vi "CS상태머신서버장난감.vi"() -> ()   [LabVIEW 2018]
uses:
  <vilib>/LabVIEW Open Source Project/Connection/Connection/Connection.lvclass
  <vilib>/LabVIEW Open Source Project/MQTT TCP Connection/MQTT_TCP/Connection/TCPConnection.lvclass
  C:/Program Files (x86)/National Instruments/LabVIEW 2018/vi.lib/LabVIEW Open Source Project/Connection/Connection/Connection.lvclass
panel:
  in  "파일 경로(대화 상자 사용)":path
  out "All Files in Dir":path[](array[path]) caption="디렉토리내의 모든 파일"
  out "문자열":string
  out "listener error":errorcluster
  out "server session error":errorcluster
  out "client connected":bool
  in  "정지":bool
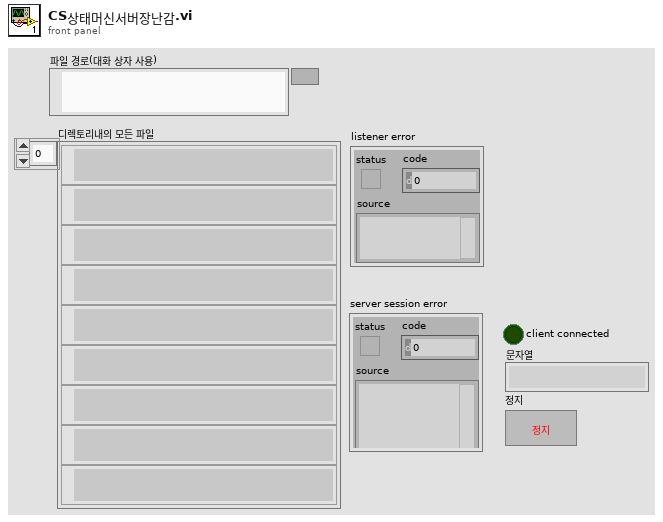
[diagram p1: front panel]
types:
  T1 = typedef "장난감컨트롤.ctl" = enum16{"대기", "연결됨", "연결종료", "종료", "업데이트", "다운로드"}
  T2 = enum16{"open", "replace", "create", "open or create", "replace or create", "replace or create with confirmation"}
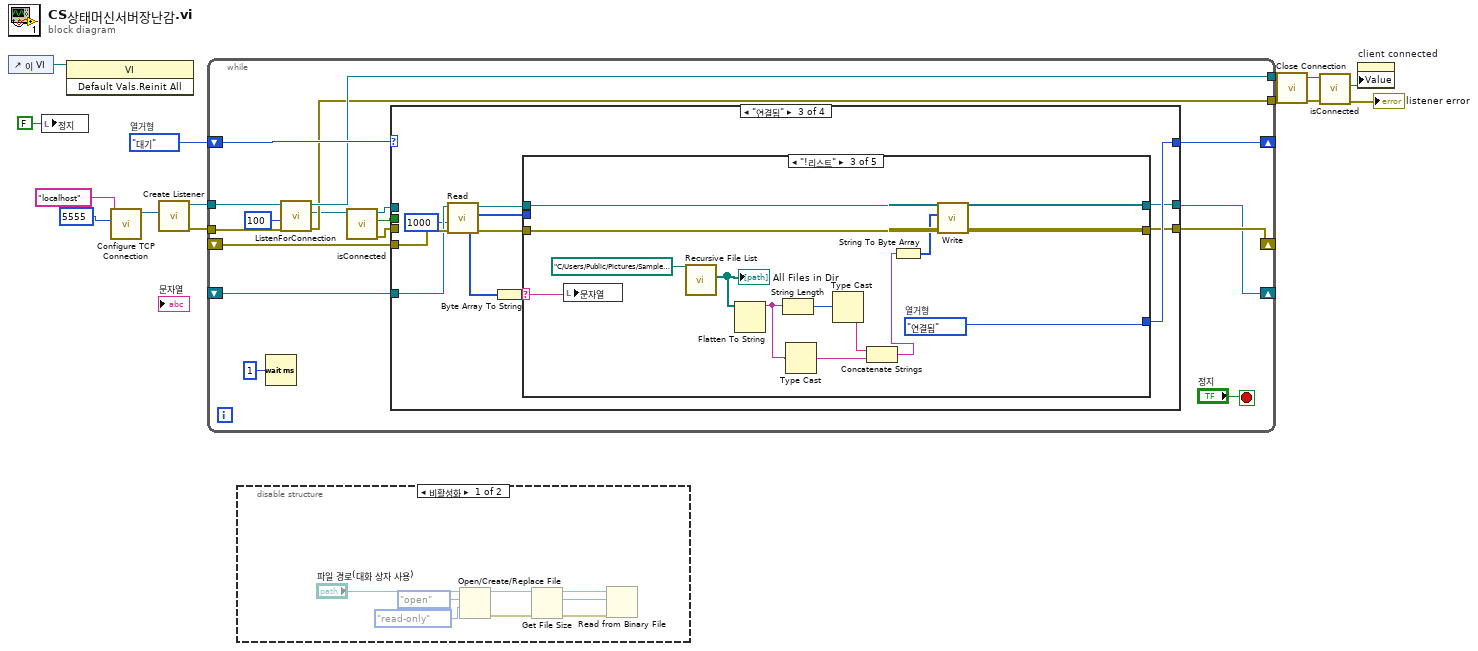
[diagram p0: block diagram]
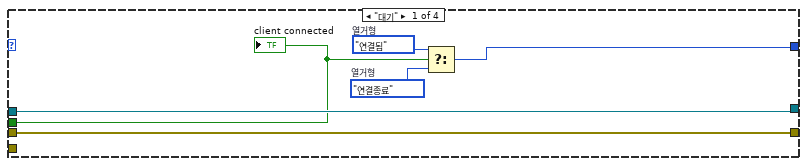
[diagram p3: hidden frame]
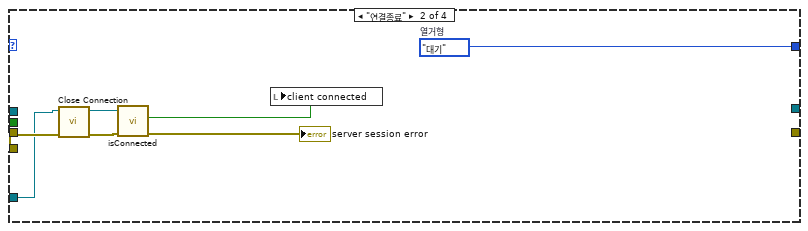
[diagram p4: hidden frame]
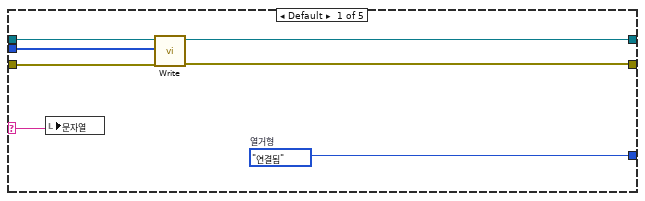
[diagram p5: hidden frame]
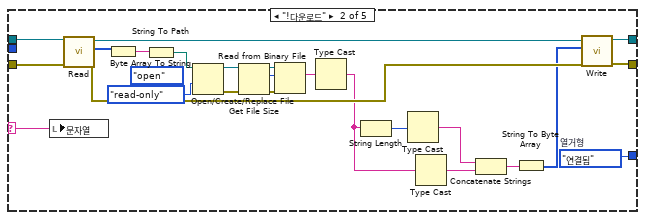
[diagram p6: hidden frame]
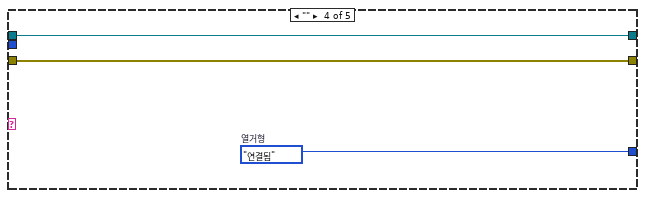
[diagram p7: hidden frame]
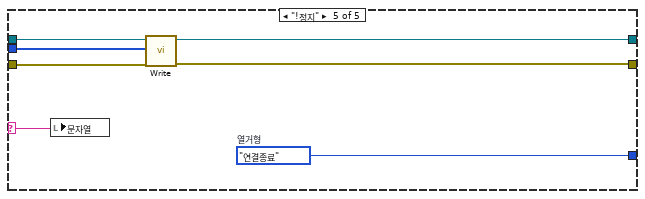
[diagram p8: hidden frame]
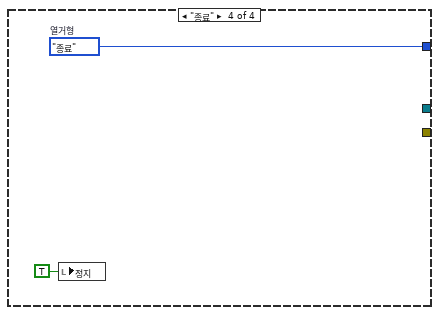
[diagram p9: hidden frame]
diagram:
  w7 = 장난감컨트롤."대기"  # 열거형
  n1 = control-ref of="이 VI"() -> (w11:refnum<vi>)
  n2 = local write "정지"(FALSE ("정지")) -> ()
  n3 = invoke class="VI" method="Default Vals.Reinit All"(reference=w11) -> ()  [unwired: 2 in, 3 out]
  n4 = call <vilib>:"Configure TCP Connection.vi"("remote port (80)"=u16 5555, "address (localhost)"="localhost") -> ("TCPConnection"=w14:refnum<class "TCPConnection.lvclass">)  [unwired: 8 in, 1 out]
  n5 = call <vilib>:"Create Listener.vi"("Connection Configuration"=w14) -> ("error out"=w6:errorcluster, "Listener"=w5:refnum<class "TCPConnection.lvclass">)  [unwired: 9 in]
  n6 = while {
    tunnel: [w27] -> w9
    tunnel: [w25] -> w8
    shift-right: [w28] -> _
    shift-left: w7 -> [w29]
    tunnel: w6 -> [w26]
    shift-right: [w24] -> _
    shift-left: _ -> [w23]
    tunnel: w5 -> [w17]
    shift-right: [w16] -> _
    shift-left: _ -> [w15]
    stop <- "정지" stop-if-true
    n7 = Wait (ms)(milliseconds to wait=u32 1 ("대기 시간 (ms)")) -> ()  [unwired: 1 out]
    n8 = call <vilib>:"ListenForConnection.vi"("error in (no error)"=w26, "timeout (2000 ms)"=100, "Listener"=w17) -> ("error out"=w25:errorcluster, "Connection"=w22:refnum<class "Connection.lvclass">, "Listener out"=w27:refnum<class "TCPConnection.lvclass">)  [unwired: 5 in, 1 out]
    n9 = call <vilib>:"isConnected.vi"("Connection in"=w22) -> ("error out"=w20:errorcluster, "connected"=w19:bool, "Connection out"=w21:refnum<class "Connection.lvclass">)  [unwired: 8 in]
    n10 = case shown="\"연결됨\"" w29 {
      tunnel: [w37 w40 w50 w111] -> w28
      tunnel: [w34 _ w46 _] -> w16
      tunnel: [w32 _ w45 _] -> w24
      tunnel: w23 -> [_ w39 w54 _]
      tunnel: w21 -> [w34 _ _ _]
      tunnel: w20 -> [w32 _ _ _]
      tunnel: w19 -> [w33 _ _ _]
      tunnel: w15 -> [_ w38 w53 _]
      frame "대기" {
        w35 = 장난감컨트롤."연결종료"  # 열거형
        w36 = 장난감컨트롤."연결됨"  # 열거형
        n11 = Select(t=w36, s=w33, f=w35) -> (s? t:f=w37:T1)
        "client connected" <- w33
      }
      frame "연결종료" {
        w40 = 장난감컨트롤."대기"  # 열거형
        n12 = call <vilib>:"Close Connection.vi"("error in (no error)"=w39, "Connection in"=w38) -> ("error out"=w41:errorcluster, "No Connection"=w43:refnum<class "Connection.lvclass">)  [unwired: 8 in]
        n13 = call <vilib>:"isConnected.vi"("error in (no error)"=w41, "Connection in"=w43) -> ("error out"=→"server session error":errorcluster, "connected"=w44:bool)  [unwired: 7 in, 1 out]
        n14 = local write "client connected"(w44) -> ()
      }
      frame "연결됨" {
        n15 = call <vilib>:"Read.vi"("error in (no error)"=w54, "timeout (2000 ms)"=1000, "TCPConnection in"=w53) -> ("error out"=w49:errorcluster, "Bytes"=w48:u8[], "TCPConnection out"=w47:refnum<class "Connection.lvclass">)  [unwired: 4 in, 2 out]
        n16 = Byte Array To String(unsigned byte array=w48) -> (string=w51:string)
        n17 = case shown="\"!리스트\"" w51 {
          selector: w51 -> [w61 w66 w99 _ w103]
          tunnel: [w60 w71 w98 w102 w109] -> w50
          tunnel: w49 -> [w59 w84 w97 w100 w106]
          tunnel: w48 -> [w58 _ _ _ w107]
          tunnel: w47 -> [w57 w85 w96 w101 w108]
          tunnel: [w56 w73 w95 w101 w104] -> w46
          tunnel: [w55 w72 w94 w100 w105] -> w45
          frame Default {
            w60 = 장난감컨트롤."연결됨"  # 열거형
            n18 = local write "문자열"(w61) -> ()
            n19 = call <vilib>:"Write.vi"("error in (no error)"=w59, "Bytes"=w58, "Connection in"=w57) -> ("error out"=w55:errorcluster, "Connection"=w56:refnum<class "Connection.lvclass">)  [unwired: 7 in]
          }
          frame "!다운로드" {
            w71 = 장난감컨트롤."연결됨"  # 열거형
            (unwired) T2."open" ("동작(0:open)")
            n20 = local write "문자열"(w66) -> ()
            n21 = call <vilib>:"Read.vi"("error in (no error)"=w84, "TCPConnection in"=w85) -> ("error out"=w74:errorcluster, "Bytes"=w83:u8[], "TCPConnection out"=w75:refnum<class "Connection.lvclass">)  [unwired: 5 in, 2 out]
            n22 = Byte Array To String(unsigned byte array=w83) -> (string=w79:string)
            n23 = String To Path(string=w79) -> (path=w78:path)
            n24 = Open/Create/Replace File(file path (use dialog)=w78, access (0:read/write)=enum16{"read/write", "read-only", "write-only"}."read-only" ("접근(0:읽기/쓰기)")) -> (refnum out=w77:refnum<file>, error out=w81:errorcluster)  [unwired: 4 in, 1 out]
            n25 = Get File Size(file=w77, error in=w81) -> (refnum out=w76:refnum<file>, size (in bytes)=w65:i64, 0:w82:errorcluster)
            n26 = Read from Binary File(8:w82, 10:w65, 11:w76) -> (2:w64:string)  [unwired: 3 in, 3 out]
            n27 = Type Cast(x=w64) -> (*(type *) &x=w62:string)  [unwired: 1 in]
            n28 = String Length(string=w62) -> (length=w63:i32)
            n29 = Type Cast(x=w63) -> (*(type *) &x=w70:string)  [unwired: 1 in]
            n30 = Type Cast(x=w62) -> (*(type *) &x=w69:string)  [unwired: 1 in]
            n31 = Concatenate Strings(w70, w69) -> (w68:string)
            n32 = String To Byte Array(string=w68) -> (unsigned byte array=w67:u8[])
            n33 = call <vilib>:"Write.vi"("error in (no error)"=w74, "Bytes"=w67, "Connection in"=w75) -> ("error out"=w72:errorcluster, "Connection"=w73:refnum<class "Connection.lvclass">)  [unwired: 7 in]
          }
          frame "!리스트" {
            w98 = 장난감컨트롤."연결됨"  # 열거형
            n34 = local write "문자열"(w99) -> ()
            n35 = call <vilib>:"Recursive File List.vi"("Folder Path"=path "C:/Users/Public/Pictures/Sample Pictures") -> ("All Files in Dir"=w91:path[])  [unwired: 6 in, 4 out]
            "All Files in Dir" <- w91
            n36 = Flatten To String(anything=w91) -> (data string=w88:string)  [unwired: 3 in, 2 out]
            n37 = String Length(string=w88) -> (length=w90:i32)
            n38 = Type Cast(x=w88) -> (*(type *) &x=w86:string)  [unwired: 1 in]
            n39 = Type Cast(x=w90) -> (*(type *) &x=w87:string)  [unwired: 1 in]
            n40 = Concatenate Strings(w87, w86) -> (w89:string)
            n41 = String To Byte Array(string=w89) -> (unsigned byte array=w92:u8[])
            n42 = call <vilib>:"Write.vi"("error in (no error)"=w97, "Bytes"=w92, "Connection in"=w96) -> ("error out"=w94:errorcluster, "Connection"=w95:refnum<class "Connection.lvclass">)  [unwired: 7 in]
          }
          frame "" {
            w102 = 장난감컨트롤."연결됨"  # 열거형
          }
          frame "!정지" {
            w109 = 장난감컨트롤."연결종료"  # 열거형
            n43 = local write "문자열"(w103) -> ()
            n44 = call <vilib>:"Write.vi"("error in (no error)"=w106, "Bytes"=w107, "Connection in"=w108) -> ("error out"=w105:errorcluster, "Connection"=w104:refnum<class "Connection.lvclass">)  [unwired: 7 in]
          }
        }
      }
      frame "종료" {
        w111 = 장난감컨트롤."종료"  # 열거형
        n45 = local write "정지"(TRUE ("정지")) -> ()
      }
    }
  }
  n46 = disable-structure shown="비활성화" {
    frame Disabled {
      n47 = Open/Create/Replace File(file path (use dialog)="파일 경로(대화 상자 사용)", operation (0:open)=T2."open" ("동작(0:open)"), access (0:read/write)=enum16{"read/write", "read-only", "write-only"}."read-only" ("접근(0:읽기/쓰기)")) -> (refnum out=w115:refnum<file>, error out=w117:errorcluster)  [unwired: 3 in, 1 out]
      n48 = Get File Size(file=w115, error in=w117) -> (refnum out=w116:refnum<file>, size (in bytes)=w119:i64, 0:w118:errorcluster)
      n49 = Read from Binary File(8:w118, 10:w119, 11:w116) -> ()  [unwired: 3 in, 4 out]
    }
    frame Enabled {
    }
  }
  n50 = call <vilib>:"Close Connection.vi"("error in (no error)"=w8, "Connection in"=w9) -> ("error out"=w4:errorcluster, "No Connection"=w3:refnum<class "TCPConnection.lvclass">)  [unwired: 8 in]
  n51 = call <vilib>:"isConnected.vi"("error in (no error)"=w4, "Connection in"=w3) -> ("error out"=→"listener error":errorcluster, "connected"=w2:bool)  [unwired: 7 in, 1 out]
  n52 = property on="client connected" class="Bool (엄격한)"("Value"=w2) -> ()  [unwired: 2 in, 2 out]
